vi "Generate Plugin Error String Array.vi"(8 "error in (no error)":errorcluster, 11 "Full Plugin Array":T1[](array[typedef])) -> (0 "error out":errorcluster, 3 "Error Strings":string[](array[string]))   [LabVIEW 2020, in "RxnRover.lvlib" / "Plugin Manager.lvlib"]
doc: "Helper VI which formats plugin error clusters and ouputs an array of formatted strings (This subVI does not write to a log file)\nWith the format;\n[Time RTC 3339] [Plugin Name] Error: Message\n[Time RTC 3339] [Plugin Name] Error: Message\n[Time RTC 3339] [Plugin Name] Error: Message\n. . .\n\nCreated 5/20/2025 - Labview 2020\nRxnRover"
uses:
  Plugin Manager.lvlib
  Plugin Details.ctl
  Plugin Servers/Controller/Controller Type.ctl
  Plugin Types.ctl
  Config Error.ctl
  Plugin Servers/Controller/Generic Plugin.lvclass
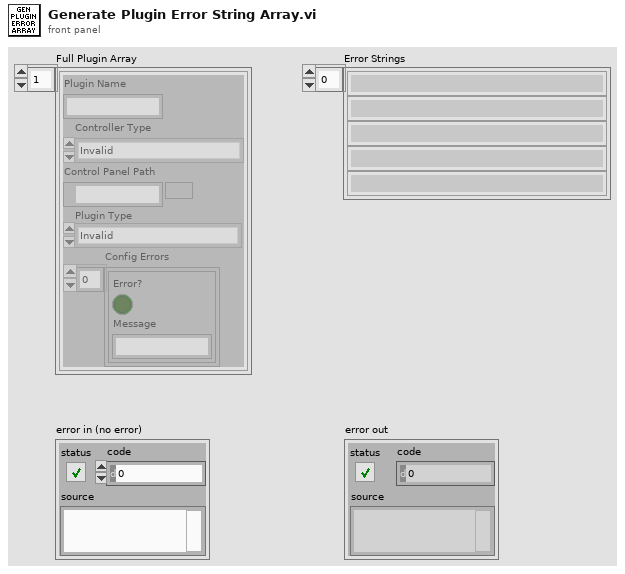
[diagram p1: front panel]
types:
  T1 = typedef "RxnRover.lvlib/Plugin Manager.lvlib/Plugin Details.ctl" = cluster{"Plugin Name":string, "Controller Type":T2, "Control Panel Path":path, "Plugin Type":T3, "Config Errors":T4[]}
  T2 = typedef "RxnRover.lvlib/Generic Plugin.lvclass/Controller Type.ctl" = enum16{"Invalid", "Temperature Controller", "Pump Controller", "Syringe Pump", "Generic Optimizer", "LC Parser", "Passive Hardware"}
  T3 = typedef "RxnRover.lvlib/Plugin Manager.lvlib/Plugin Types.ctl" = enum16{"Invalid", "Optimizer", "Analyzer", "Hardware"}
  T4 = typedef "RxnRover.lvlib/Plugin Manager.lvlib/Config Error.ctl" = cluster{"Error?":bool, "Message":string}
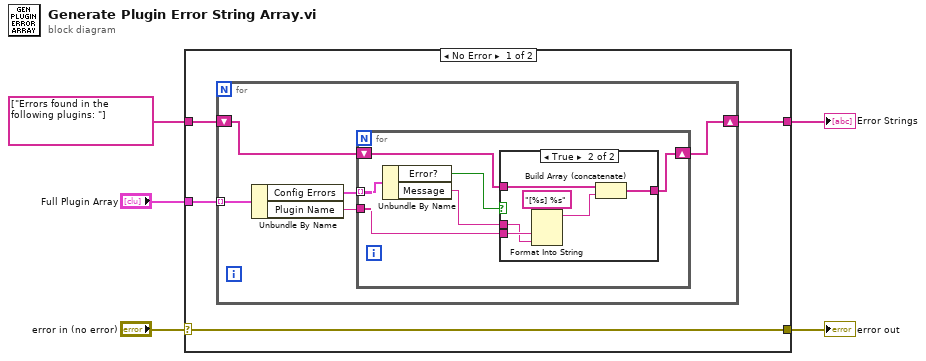
[diagram p0: block diagram]
diagram:
  n1 = case shown="No Error" "error in (no error)" {
    selector: "error in (no error)" -> [w6 w28]
    tunnel: [w9 w29] -> w5
    tunnel: string[] ["Errors found in the following plugins: "] -> [w8 w29]
    tunnel: "Full Plugin Array" -> [w7 _]
    tunnel: [w6 w28] -> w1
    frame No Error {
      n2 = for {
        tunnel: w7 -> [w14] mode=indexing
        shift-right: [w11] -> w9
        shift-left: w8 -> [w10]
        n3 = Unbundle By Name(w14) -> ("Config Errors"=w13:T4[], "Plugin Name"=w12:string)
        n4 = for {
          tunnel: w13 -> [w20] mode=indexing
          tunnel: w12 -> [w17]
          shift-right: [w15] -> w11
          shift-left: w10 -> [w19]
          n5 = Unbundle By Name(w20) -> ("Error?"=w18:bool, "Message"=w16:string)
          n6 = case shown="True" w18 {
            tunnel: w19 -> [w21 w27]
            tunnel: w17 -> [_ w25]
            tunnel: w16 -> [_ w24]
            tunnel: [w21 w22] -> w15
            frame False {
            }
            frame True {
              n7 = Format Into String(format string="[%s] %s", w25, w24) -> (resulting string=w23:string)  [unwired: 2 in, 1 out]
              n8 = Build Array (concatenate)(w27, w23) -> (w22:string[])
            }
          }
        }
      }
    }
    frame Error {
    }
  }
  "Error Strings" <- w5
  "error out" <- w1
